vi "GitSetup.vi"(8 "error in (no error)":errorcluster, 9 "Directory":path=path "", 11 "Git exec":string="git") -> (0 "error out":errorcluster, 1 "Directory out":path, 2 "Response":string, 3 "Git exec out":string="git")   [LabVIEW 2013]
uses:
  GitCmd.vi
  <vilib>/dlg_ctls.llb/Space Constant.vi
  GitUtils/PathtoDirPath.vi
  <vilib>/Platform/system.llb/System Exec.vi
  <vilib>/Utility/error.llb/Error Cluster From Error Code.vi
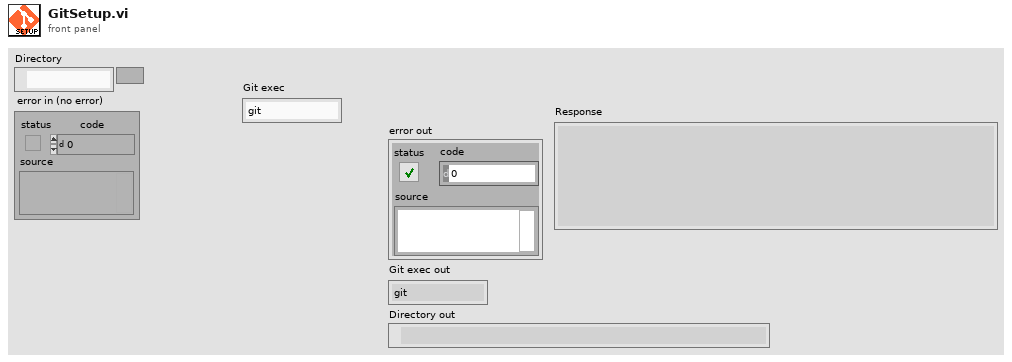
[diagram p1: front panel]
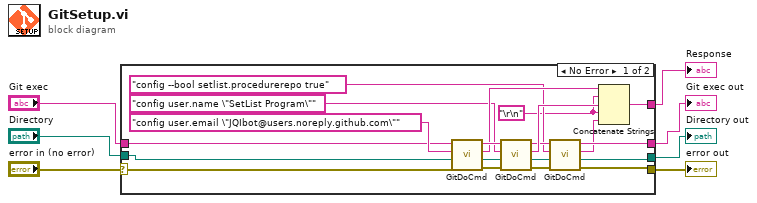
[diagram p0: block diagram]
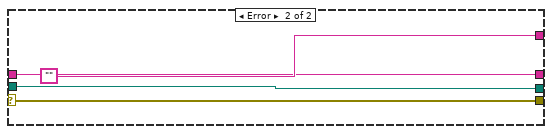
[diagram p2: hidden frame]
diagram:
  n1 = case shown="No Error" "error in (no error)" {
    selector: "error in (no error)" -> [w22 w30]
    tunnel: "Git exec" -> [w20 w28]
    tunnel: "Directory" -> [w21 w29]
    tunnel: [w27 ""] -> w5
    tunnel: [w15 w30] -> w4
    tunnel: [w14 w29] -> w2
    tunnel: [w12 w28] -> w1
    frame No Error {
      w9 = "\r\n"
      n2 = call "GitDoCmd.vi"("error in (no error)"=w22, "Working Path"=w21, "Git command"="config user.email \"JQIbot@users.noreply.github.com\"" ("string"), "Git exec"=w20) -> ("error out"=w23:errorcluster, "Working Path out"=w24:path, "Returned stdout"=w19:string, "Git exec out"=w26:string)  [unwired: 3 in]
      n3 = call "GitDoCmd.vi"("error in (no error)"=w23, "Working Path"=w24, "Git command"="config user.name \"SetList Program\"" ("string"), "Git exec"=w26) -> ("error out"=w17:errorcluster, "Working Path out"=w16:path, "Returned stdout"=w18:string, "Git exec out"=w13:string)  [unwired: 3 in]
      n4 = call "GitDoCmd.vi"("error in (no error)"=w17, "Working Path"=w16, "Git command"="config --bool setlist.procedurerepo true" ("string"), "Git exec"=w13) -> ("error out"=w15:errorcluster, "Working Path out"=w14:path, "Returned stdout"=w10:string, "Git exec out"=w12:string)  [unwired: 3 in]
      n5 = Concatenate Strings(w19, w9, w18, w9, w10) -> (w27:string)
    }
    frame Error {
    }
  }
  "Response" <- w5
  "error out" <- w4
  "Git exec out" <- w1
  "Directory out" <- w2
